vi "setChannelDefaults.vi"(8 "error in (no error)":errorcluster, 9 "Data":variant, 10 "physicalChannels":string[](array[string]), 11 "DDSOutput in":refnum<class "DDSOutput.lvclass">) -> (0 "error out":errorcluster, 3 "DDSOutput out":refnum<class "DDSOutput.lvclass">)   [LabVIEW 2011, in "Hardware.lvlib" / "Channels.lvlib" / "DDSOutput.lvclass"]
doc: "Default Data Cluster:\n\n1) frequency (db)\n2) amplitude (db)\n3) phase (db)\n4) type (enum: sine, square, triangle)"
uses:
  DDSOutput.lvclass
  DDSOutput.lvclass/DDSOutput.ctl
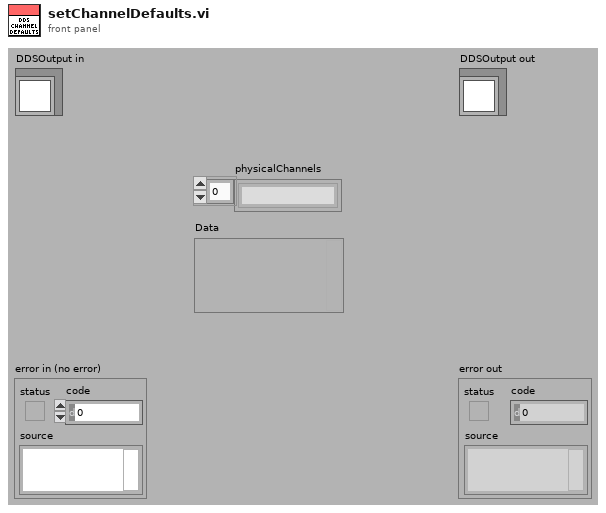
[diagram p1: front panel]
types:
  T1 = cluster{dbl, "Amplitude":dbl, "Phase":dbl, "OutputForm":enum16{"Sine", "Square", "Triangle", "Arbitrary"}}[]
  T2 = cluster{"Frequency(MHz)":dbl, "Amplitude":dbl, "Phase":dbl, "OutputForm":enum16{"Sine", "Square", "Triangle", "Arbitrary"}}[]
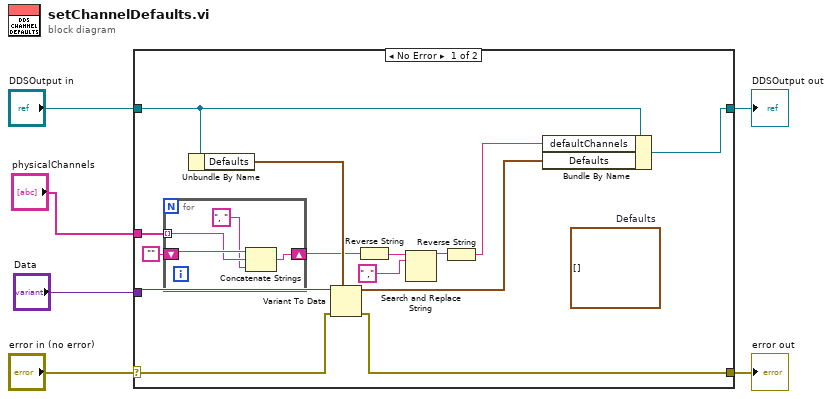
[diagram p0: block diagram]
diagram:
  n1 = case shown="No Error" "error in (no error)" {
    selector: "error in (no error)" -> [w16 w26]
    tunnel: [w15 w26] -> w5
    tunnel: [w20 w25] -> w3
    tunnel: "DDSOutput in" -> [w19 w25]
    tunnel: "Data" -> [w18 _]
    tunnel: "physicalChannels" -> [w13 _]
    frame No Error {
      (unwired) T1 []  # Defaults
      n2 = for {
        tunnel: w13 -> [w23] mode=indexing
        shift-right: [w21] -> w11
        shift-left: "" -> [w24]
        n3 = Concatenate Strings(w24, w23, ", ") -> (w21:string)
      }
      n4 = Unbundle By Name(w19) -> ("Defaults"=w17:T2)
      n5 = Variant To Data(error in=w16, type=w17, Variant=w18) -> (data=w14:T2, error out=w15:errorcluster)
      n6 = Reverse String(1:w11) -> (0:w10:string)
      n7 = Search and Replace String(input string=w10, search string=" ,") -> (result string=w8:string)  [unwired: 6 in, 3 out]
      n8 = Reverse String(1:w8) -> (0:w7:string)
      n9 = Bundle By Name(cluster=w19, "defaultChannels"=w7, "Defaults"=w14) -> (w20:refnum<class "DDSOutput.lvclass">)
    }
    frame Error {
    }
  }
  "error out" <- w5
  "DDSOutput out" <- w3
